vi "animate options opening.vi"(7 "Top Splitter in":refnum<vi>, 10 "expand/collapse":bool, 11 "Bottom Splitter in":refnum<vi>) -> ()   [LabVIEW 2016, in "RM.Server.lvlib"]
uses:
  RM.Server.lvlib
  Shared/Global Tags.vi
  Shared/RM.Shared.lvlib
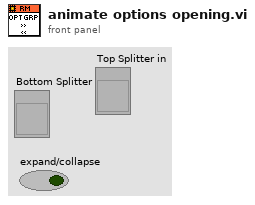
[diagram p1: front panel]
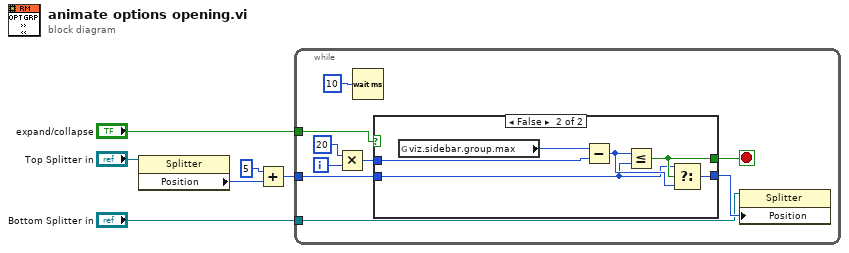
[diagram p0: block diagram]
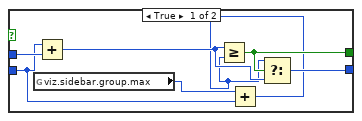
[diagram p2: hidden frame]
diagram:
  n1 = property on="Property Node" class="Splitter"(reference="Top Splitter in") -> ("Position"=w3:i32)  [unwired: 1 in, 2 out]
  n2 = Add(x=5, y=w3) -> (x+y=w2:i32)
  n3 = while {
    tunnel: "expand/collapse" -> [w15]
    tunnel: "Bottom Splitter in" -> [w8]
    tunnel: w2 -> [w7]
    i -> [w11]
    stop <- w14 stop-if-true
    n4 = Multiply(x=20, y=w11) -> (x*y=w10:i32)
    n5 = Wait (ms)(milliseconds to wait=u32 10) -> ()  [unwired: 1 out]
    n6 = case shown="False" w15 {
      tunnel: [w21 w26] -> w14
      tunnel: [w19 w24] -> w13
      tunnel: w10 -> [w22 w28]
      tunnel: w7 -> [w16 w23]
      frame True {
        n7 = global read "Global Tags.vi" "viz.sidebar.group.max"() -> (w18:i32)
        n8 = Add(x=w16, y=w22) -> (x+y=w20:i32)
        n9 = Add(x=w18, y=w16) -> (x+y=w17:i32)
        n10 = Greater Or Equal?(x=w20, y=w17) -> (x >= y?=w21:bool)
        n11 = Select(t=w17, s=w21, f=w20) -> (s? t:f=w19:i32)
      }
      frame False {
        n12 = global read "Global Tags.vi" "viz.sidebar.group.max"() -> (w27:i32)
        n13 = Subtract(x=w27, y=w28) -> (x-y=w25:i32)
        n14 = Less Or Equal?(x=w25, y=w23) -> (x <= y?=w26:bool)
        n15 = Select(t=w23, s=w26, f=w25) -> (s? t:f=w24:i32)
      }
    }
    n16 = property on="Property Node" class="Splitter"(reference=w8, "Position"=w13) -> ()  [unwired: 1 in, 2 out]
  }
